vi "inteference -- find center V24.vi"(6 "weights":dbl[](array[numeric]), 7 "number of points":i32, 8 "complex region":T1={"max re"=5.161869466666667e-06, "min re"=5.176843333333334e-06, "max im"=-2.467216e-05, "min im"=-0.001573233, "delta re"=0.003211203, "delta im"=0.00165815, "center re"=0.0015485608400000002, "delta  z"=0.0015530530000000002+0.0i, "center im"=0.0, "center z"=0.0+0.0i, "d im"=0.0, "d re"=0.0, "d z"=0.0+0.0i}, 9 "pond":cdb[][](array[numeric]), 10 "point sources":cdb[](array[numeric]), 11 "wave packet":cdb[][](array[numeric])) -> (2 "z (center)":cdb)   [LabVIEW 2018]
uses:
  complex region.ctl
  <vilib>/Analysis/baseanly.llb/A x B.vi
  <vilib>/Analysis/baseanly.llb/Real A x B.vi
  <vilib>/Analysis/baseanly.llb/Mean.vi
  <vilib>/Analysis/baseanly.llb/Mean (DBL).vi
  <vilib>/Analysis/Matrix/Numeric/Conversions/Array To Matrix - CA2.vi
  <vilib>/Analysis/Matrix/Numeric/Multiply/Multiply - C,CM.vi
  <vilib>/Analysis/Matrix/Numeric/Add/Add - CM,CM.vi
  <vilib>/Analysis/Matrix/Numeric/Complex/Complex To Polar - CM.vi
  <vilib>/Analysis/Matrix/NI_Matrix.lvlib
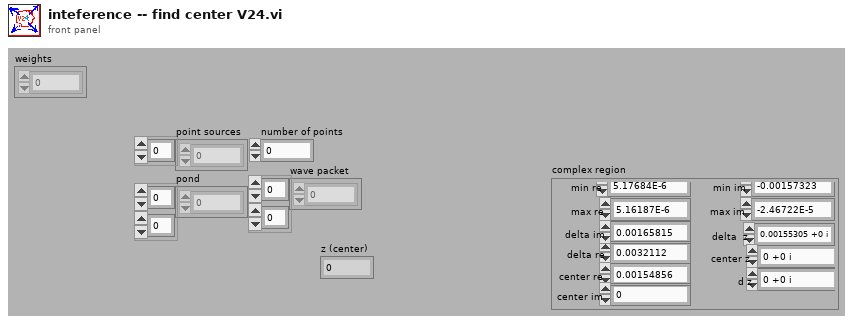
[diagram p1: front panel]
types:
  T1 = typedef "complex region.ctl" = cluster{"max re":dbl, "min re":dbl, "max im":dbl, "min im":dbl, "delta re":dbl, "delta im":dbl, "center re":dbl, "delta  z":cdb, "center im":dbl, "center z":cdb, "d im":dbl, "d re":dbl, "d z":cdb}
  T2 = typedef "NI_Matrix.lvlib/ComplexMatrix.ctl" = cdb[][]
  T3 = typedef "NI_Matrix.lvlib/RealMatrix.ctl" = dbl[][]
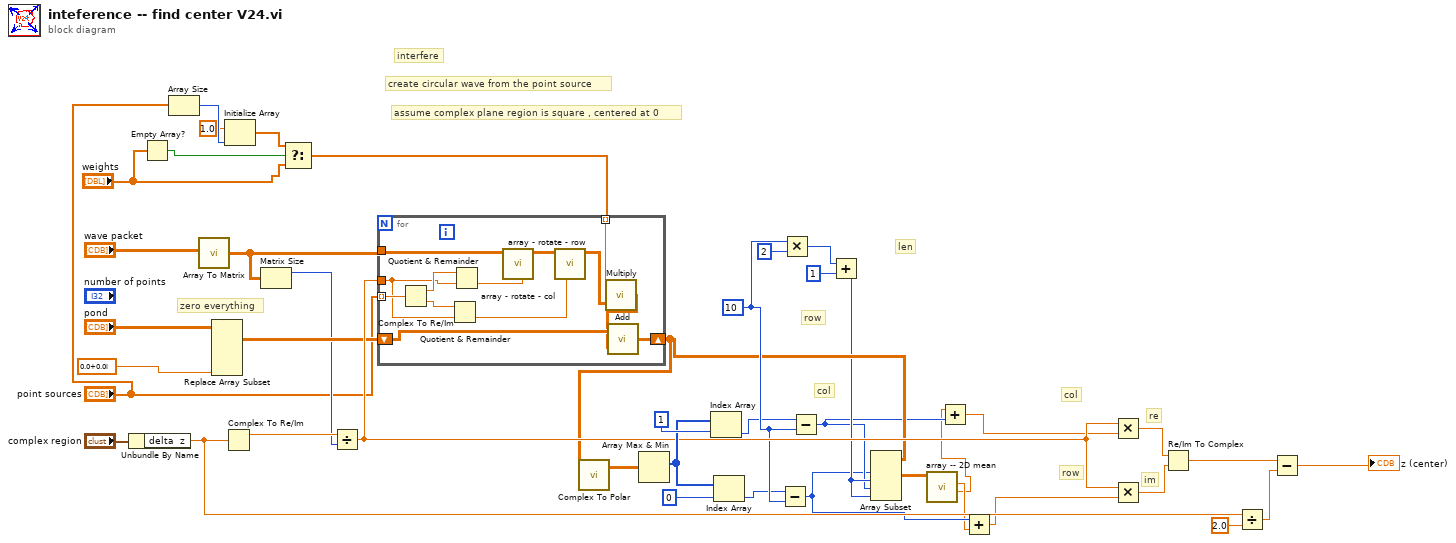
[diagram p0: block diagram]
diagram:
  w15 = 10 ("index")
  # "col"
  # "row"
  # "col"
  # "len"
  # "row"
  # "interfere"
  # "create circular wave from the point source"
  # "zero everything"
  # "assume complex plane region is square , centered at 0"
  # "re"
  # "im"
  n1 = Unbundle By Name("complex region") -> ("delta  z"=w33:cdb)
  n2 = Empty Array?(array="weights") -> (empty?=w19:bool)
  n3 = Array Size(array="point sources") -> (size(s)=w21:i32)
  n4 = call-poly <vilib>:"Array To Matrix.vi"("Complex 2D Array"="wave packet") -> ("Complex Matrix"=w24:T2)
  n5 = Replace Array Subset(array="pond", new element=cdb 0.0+0.0i) -> (w26:T2)  [unwired: 4 in]
  n6 = Complex To Re/Im(x + iy=w33) -> (x=w37:dbl)  [unwired: 1 out]
  n7 = Initialize Array(1.0 ("element"), w21) -> (w18:dbl[])
  n8 = Matrix Size(0:w24) -> (1:w23:i32)  [unwired: 1 out]
  n9 = Select(t=w18, s=w19, f="weights") -> (s? t:f=w16:dbl[])
  n10 = Divide(x=w37, y=w23) -> (x/y=w29:dbl)
  n11 = for {
    shift-right: [w54] -> w11
    shift-left: w26 -> [w55]
    tunnel: "point sources" -> [w51] mode=indexing
    tunnel: w24 -> [w49]
    tunnel: w29 -> [w50]
    tunnel: w16 -> [w45] mode=indexing
    n12 = Complex To Re/Im(x + iy=w51) -> (x=w53:dbl, y=w52:dbl)
    n13 = Quotient & Remainder(x=w52, y=w50) -> (floor(x/y)=w46:dbl)  [unwired: 1 out]
    n14 = Quotient & Remainder(x=w53, y=w50) -> (floor(x/y)=w47:dbl)  [unwired: 1 out]
    n15 = call "array - rotate - col.vi"("rotate column"=w47, "input matrix"=w49) -> ("output matrix"=w48:T2)  [unwired: 9 in]
    n16 = call "array - rotate - row.vi"("rotate row"=w46, "input matrix"=w48) -> ("output matrix"=w44:T2)  [unwired: 9 in]
    n17 = call-poly <vilib>:"Multiply.vi"("Complex Matrix A"=w44, "Complex Scalar c"=w45) -> ("c * A"=w43:T2)
    n18 = call-poly <vilib>:"Add.vi"("Complex Matrix B"=w43, "Complex Matrix A"=w55) -> ("A + B"=w54:T2)
  }
  n19 = call-poly <vilib>:"Complex To Polar.vi"("Complex Matrix r*e^iQ"=w11) -> ("Modulus r"=w39:T3)  [unwired: 1 out]
  n20 = Array Max & Min(array=w39) -> (max index (indices)=w38:i32[])  [unwired: 3 out]
  n21 = Index Array(array=w38, index=1) -> (element=w7:i32)
  n22 = Index Array(array=w38, index=0) -> (element=w8:i32)
  n23 = Subtract(x=w8, y=w15) -> (x-y=w4:i32)
  n24 = Multiply(x=w15, y=2) -> (x*y=w13:i32)
  n25 = Subtract(x=w7, y=w15) -> (x-y=w6:i32)
  n26 = Add(x=w13, y=1) -> (x+y=w10:i32)
  n27 = Array Subset(array=w11, index (row)=w4, length (row)=w10, index (col)=w6, length (col)=w10) -> (w9:T2)
  n28 = call "array -- 2D mean .vi"("pond"=w9) -> ("mean row"=w1:dbl, "mean col"=w2:dbl)  [unwired: 9 in]
  n29 = Add(x=w1, y=w6) -> (x+y=w5:dbl)
  n30 = Add(x=w4, y=w2) -> (x+y=w3:dbl)
  n31 = Multiply(x=w29, y=w5) -> (x*y=w36:dbl)
  n32 = Multiply(x=w29, y=w3) -> (x*y=w35:dbl)
  n33 = Re/Im To Complex(1:w35, 2:w36) -> (0:w31:cdb)
  n34 = Divide(x=w33, y=2.0) -> (x/y=w32:cdb)
  n35 = Subtract(x=w31, y=w32) -> (x-y=→"z (center)":cdb)
